vi "Initiate Source And Load Sequence And Wait.vi"(8 "error in (no error)":errorcluster, 11 "Reference values":T1={"dcpower session reservation"=refnum, "Source handle array"=[], "Source channel name array"=[], "Load handle"="", "Load channel name"="", "Source voltage values"=[], "Load current values"=[], "Number of steps"=0, "Source sequence name"="", "Source terminal name"="", "Measure terminal name"="", "scope session reservation"=refnum, "Scope handles"=[], "connection map"={}, "instrument info map array"=[], "Enable TClk"=FALSE, "dmm session reservation"=refnum, "dmm handle array"=[], "DMM Trigger Source"=enum."Immediate", "DMM Sample Trigger"=enum."TTL 0", "Measurement Results"={"Status"="", "Voltage values"=[], "Source sweep points"=0, "Load sweep points"=0, "Source voltages"=[], "Source currents"=[], "Load voltages"=[], "Load currents"=[], "Load voltage deviation"=[], "Efficiency"=[], "Maximum efficiency"=[], "Minimum load voltage"=[], "Maximum load voltage"=[], "Minimum load regulation"=[], "Maximum load regulation"=[], "waveform pins"=[], "waveform sites"=[], "waveform t0 array"=[], "waveform dt array"=[], "waveform length array"=[], "concatenated waveform Y"=[]}, "Additional measurements"={"voltage measurements from all sources"=[], "current measurements from all sources"=[], "all dmm measurements"=[], "all scope waverforms"=[]}}) -> (0 "error out":errorcluster, 3 "Reference values out":T1={"dcpower session reservation"=refnum, "Source handle array"=[], "Source channel name array"=[], "Load handle"="", "Load channel name"="", "Source voltage values"=[], "Load current values"=[], "Number of steps"=0, "Source sequence name"="", "Source terminal name"="", "Measure terminal name"="", "scope session reservation"=refnum, "Scope handles"=[], "connection map"={}, "instrument info map array"=[], "Enable TClk"=FALSE, "dmm session reservation"=refnum, "dmm handle array"=[], "DMM Trigger Source"=enum."Immediate", "DMM Sample Trigger"=enum."TTL 0", "Measurement Results"={"Status"="", "Voltage values"=[], "Source sweep points"=0, "Load sweep points"=0, "Source voltages"=[], "Source currents"=[], "Load voltages"=[], "Load currents"=[], "Load voltage deviation"=[], "Efficiency"=[], "Maximum efficiency"=[], "Minimum load voltage"=[], "Maximum load voltage"=[], "Minimum load regulation"=[], "Maximum load regulation"=[], "waveform pins"=[], "waveform sites"=[], "waveform t0 array"=[], "waveform dt array"=[], "waveform length array"=[], "concatenated waveform Y"=[]}, "Additional measurements"={"voltage measurements from all sources"=[], "current measurements from all sources"=[], "all dmm measurements"=[], "all scope waverforms"=[]}})   [LabVIEW 2021, in "Efficiency And Load Regulation with Pin Map.lvlib"]
uses:
  Efficiency And Load Regulation with Pin Map.lvlib
  Reference values.ctl
  <vilib>/Plug-In SDKs/Clients/Session Management V1/Session Reservation/Session Reservation.lvclass
  common/Instrument Control/Scope/TClk/Instrument Info.ctl
  common/Instrument Control/Scope Parameters.ctl
  <instrlib>/niScope/Controls/niScope vertical coupling.ctl
  <instrlib>/niDMM/nidmm.llb/niDMM Trigger.ctl
  <instrlib>/niDMM/nidmm.llb/niDMM Sample Trigger.ctl
  Measurement Results.ctl
  Additional measurements.ctl
  <instrlib>/niDCPower/nidcpower.llb/niDCPower Wait For Event - Event.ctl
  common/PMIC Common.lvlib
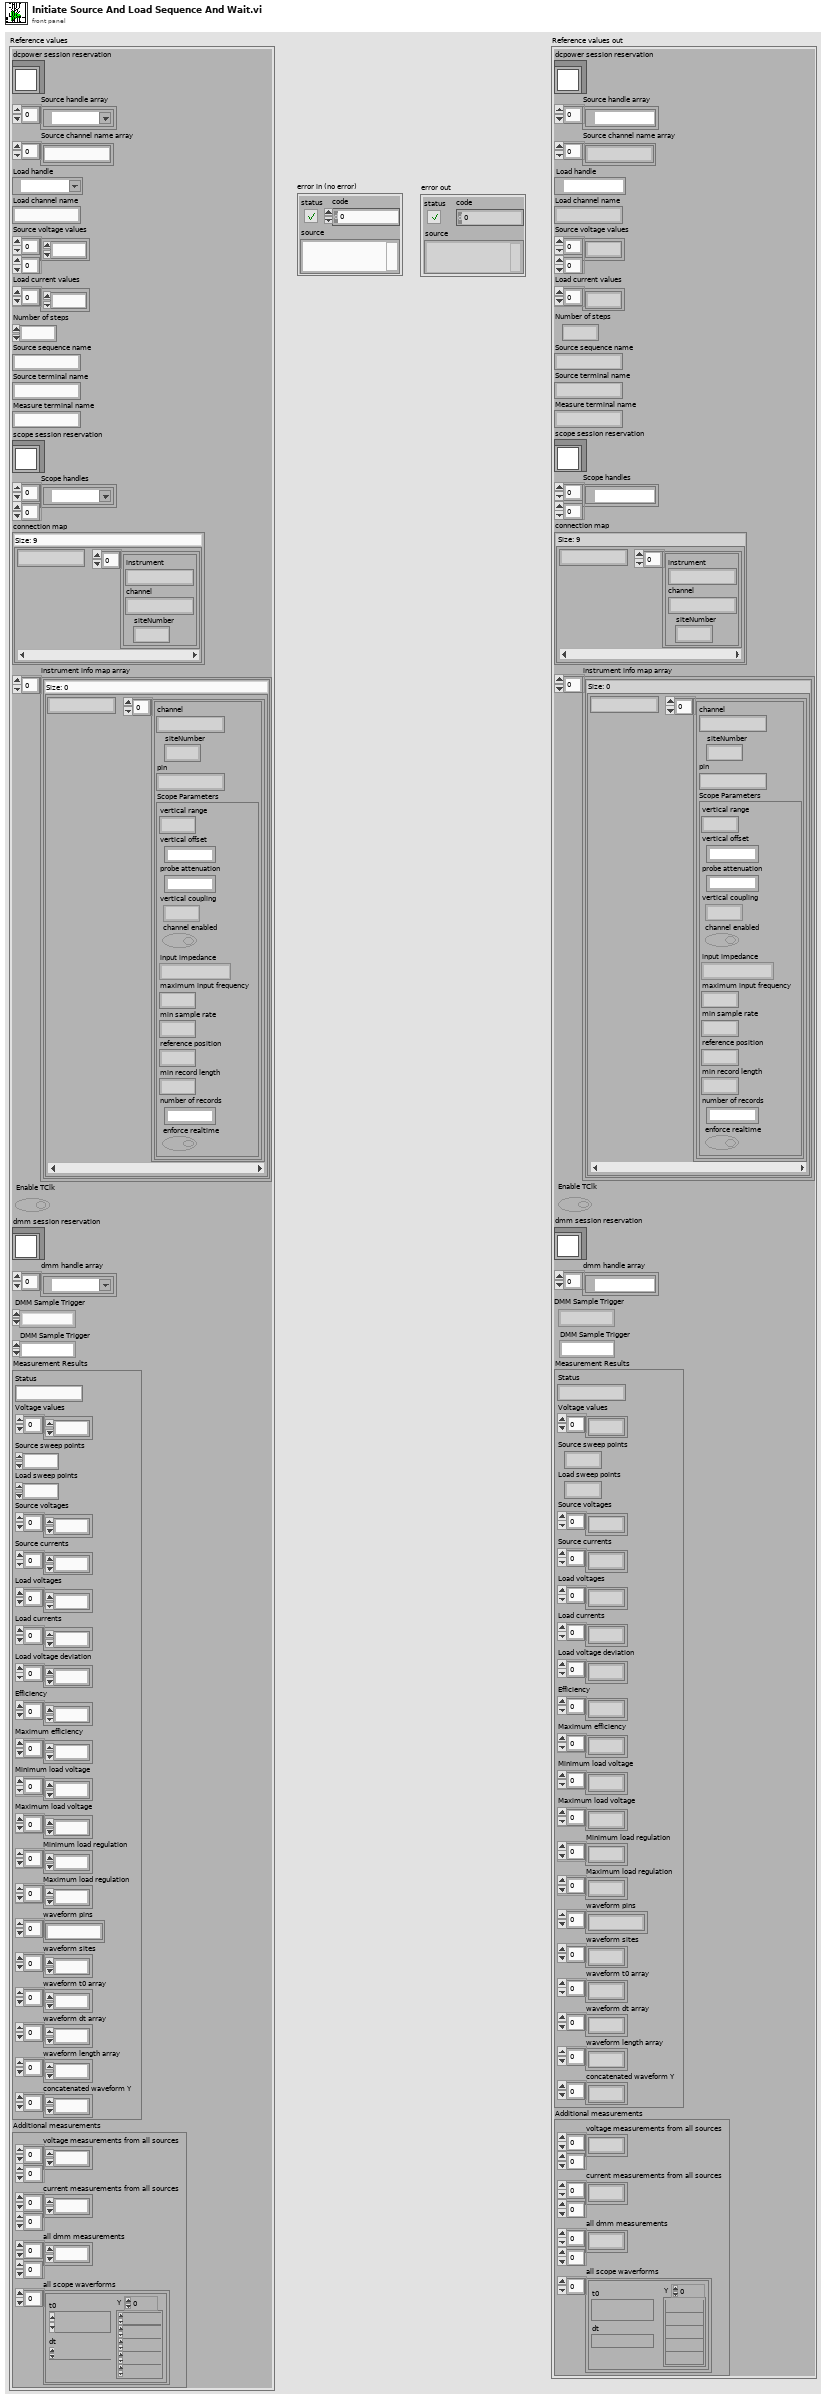
[diagram p1: front panel]
types:
  T1 = typedef "Efficiency And Load Regulation with Pin Map.lvlib/Reference values.ctl" = cluster{"dcpower session reservation":refnum<class "Session Reservation.lvclass">, "Source handle array":refnum<k15>[], "Source channel name array":string[], "Load handle":refnum<k15>, "Load channel name":string, "Source voltage values":dbl[][], "Load current values":dbl[], "Number of steps":i32, "Source sequence name":string, "Source terminal name":string, "Measure terminal name":string, "scope session reservation":refnum<class "Session Reservation.lvclass">, "Scope handles":refnum<k15>[][], "connection map":map{string, T2[]}, "instrument info map array":map{string, cluster{"channel":string, "siteNumber":i32, "pin":string, "Scope Parameters":T3}[]}[], "Enable TClk":bool, "dmm session reservation":refnum<class "Session Reservation.lvclass">, "dmm handle array":refnum<k15>[], "DMM Trigger Source":T5, "DMM Sample Trigger":T6, "Measurement Results":T7, "Additional measurements":T8}
  T2 = typedef "PMIC Common.lvlib/Instrument Info.ctl" = cluster{"instrument":string, "channel":string, "siteNumber":i32}
  T3 = typedef "PMIC Common.lvlib/Scope Parameters.ctl" = cluster{"vertical range":dbl, "vertical offset":dbl, "probe attenuation":dbl, "vertical coupling":T4, "channel enabled":bool, "input impedance":u32, "maximum input frequency":dbl, "min sample rate":dbl, "reference position":dbl, "min record length":i32, "number of records":i32, "enforce realtime":bool}
  T4 = typedef "niScope vertical coupling.ctl" = i32
  T5 = typedef "niDMM Trigger.ctl" = enum16{"Immediate", "External", "TTL 0", "TTL 1", "TTL 2", "TTL 3", "TTL 4", "TTL 5", "TTL 6", "Software", "TTL 7", "PXI Star", "LBR Trig 1", "Aux Trig 1"}
  T6 = typedef "niDMM Sample Trigger.ctl" = enum16{"Immediate", "External", "TTL 0", "TTL 1", "TTL 2", "TTL 3", "TTL 4", "TTL 5", "TTL 6", "Interval", "Software", "TTL 7", "PXI Star", "LBR Trig 1", "Aux Trig 1"}
  T7 = typedef "Efficiency And Load Regulation with Pin Map.lvlib/Measurement Results.ctl" = cluster{"Status":string, "Voltage values":dbl[], "Source sweep points":i32, "Load sweep points":i32, "Source voltages":dbl[], "Source currents":dbl[], "Load voltages":dbl[], "Load currents":dbl[], "Load voltage deviation":dbl[], "Efficiency":dbl[], "Maximum efficiency":dbl[], "Minimum load voltage":dbl[], "Maximum load voltage":dbl[], "Minimum load regulation":dbl[], "Maximum load regulation":dbl[], "waveform pins":string[], "waveform sites":i32[], "waveform t0 array":dbl[], "waveform dt array":dbl[], "waveform length array":i32[], "concatenated waveform Y":dbl[]}
  T8 = typedef "Efficiency And Load Regulation with Pin Map.lvlib/Additional measurements.ctl" = cluster{"voltage measurements from all sources":dbl[][], "current measurements from all sources":dbl[][], "all dmm measurements":dbl[][], "all scope waverforms":waveform(dbl)[]}
  T9 = typedef "niDCPower Wait For Event - Event.ctl" = i32
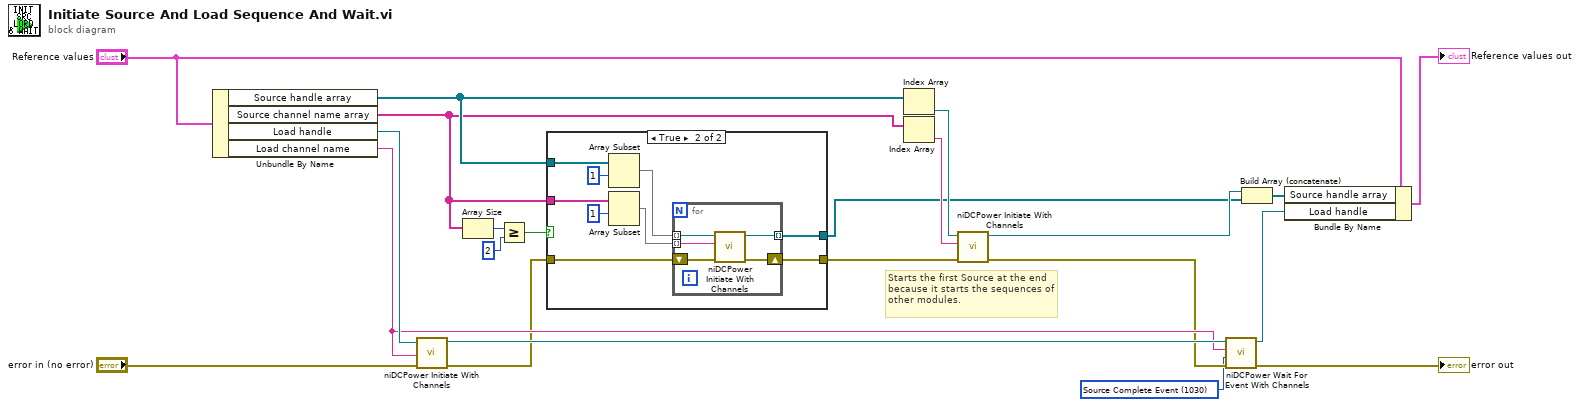
[diagram p0: block diagram]
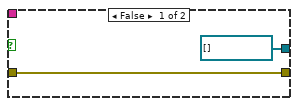
[diagram p2: hidden frame]
diagram:
  w1 = T9 1030 items=["Source Complete Event"=1030, "Measure Complete Event"=1031, "Sequence Iteration Complete Event"=1032, "Sequence Engine Done Event"=1033] ("event")
  # "Starts the first Source at the end because it starts the sequences of other modules."
  n1 = Unbundle By Name("Reference values") -> ("Source handle array"=w15:refnum<k15>[], "Source channel name array"=w12:string[], "Load handle"=w21:refnum<k15>, "Load channel name"=w20:string)
  n2 = call <instrlib>:"niDCPower Initiate With Channels.vi"("error in (no error)"="error in (no error)", "channel name"=w20, "instrument handle"=w21) -> ("error out"=w18:errorcluster, "instrument handle out"=w22:refnum<k15>)  [unwired: 7 in]
  n3 = Array Size(array=w12) -> (size(s)=w11:i32)
  n4 = Greater Or Equal?(x=w11, y=2) -> (x >= y?=w9:bool)
  n5 = case shown="True" w9 {
    tunnel: w18 -> [w24 w33]
    tunnel: [w24 w28] -> w17
    tunnel: w15 -> [_ w27]
    tunnel: w12 -> [_ w26]
    tunnel: [refnum<k15>[] [] w25] -> w4
    frame False {
    }
    frame True {
      n6 = Array Subset(array=w27, index=1) -> (w30:refnum<k15>[])  [unwired: 1 in]
      n7 = Array Subset(array=w26, index=1) -> (w29:string[])  [unwired: 1 in]
      n8 = for {
        shift-right: [w38] -> w28
        shift-left: w33 -> [w37]
        tunnel: w30 -> [w36] mode=indexing
        tunnel: w29 -> [w35] mode=indexing
        tunnel: [w34] -> w25 mode=indexing
        n9 = call <instrlib>:"niDCPower Initiate With Channels.vi"("error in (no error)"=w37, "channel name"=w35, "instrument handle"=w36) -> ("error out"=w38:errorcluster, "instrument handle out"=w34:refnum<k15>)  [unwired: 7 in]
      }
    }
  }
  n10 = Index Array(array=w15) -> (element=w14:refnum<k15>)  [unwired: 1 in]
  n11 = Index Array(array=w12) -> (element=w13:string)  [unwired: 1 in]
  n12 = call <instrlib>:"niDCPower Initiate With Channels.vi"("error in (no error)"=w17, "channel name"=w13, "instrument handle"=w14) -> ("error out"=w16:errorcluster, "instrument handle out"=w5:refnum<k15>)  [unwired: 7 in]
  n13 = call <instrlib>:"niDCPower Wait For Event With Channels.vi"("error in (no error)"=w16, "event"=w1, "channel name"=w20, "instrument handle"=w22) -> ("error out"=→"error out":errorcluster, "instrument handle out"=w19:refnum<k15>)  [unwired: 6 in]
  n14 = Build Array (concatenate)(w5, w4) -> (w6:refnum<k15>[])
  n15 = Bundle By Name(cluster="Reference values", "Source handle array"=w6, "Load handle"=w19) -> (→"Reference values out":T1)
